vi "Example UI.TestLauncher.vi"() -> ()   [LabVIEW 2016, in "Instrument.PPMS2 UI.lvclass"]
doc: "JKI State Machine Objects (SMO) 1.0.0.5\nJKI - JKI\nCopyright (c) 2016, JKI"
uses:
  Instrument.PPMS2 UI.lvclass
  C:/Program Files (x86)/National Instruments/LabVIEW 2016/vi.lib/JKI/JKI SMO/SMO/SMO.lvclass
  C:/Program Files (x86)/National Instruments/LabVIEW 2016/vi.lib/JKI/JKI SMO/SMO.UI/SMO.UI.lvclass
  instrument.PPMS2/instrument.PPMS2.lvclass
  C:/Program Files (x86)/National Instruments/LabVIEW 2016/user.lib/LevyLab/Levylab Instruments/SMOs/Instrument/Instrument.lvclass
  <vilib>/JKI/JKI SMO/SMO/Typedefs/SMOState --Enum.ctl
  <vilib>/JKI/JKI SMO/SMO/SMO.lvclass
  <vilib>/JKI/JKI SMO/SMO.UI/SMO.UI.lvclass
panel:
  out "error out":errorcluster
  in  "Stop":bool
  # "SMO UI Test Launcher"
  # "For instructions on how to use the JKI State Machine Objects, examples and video tutorials, visit:\nhttp://jki.net/state-machine-objects/\n\nJKI State Machine Objects™\nhttp://jki.net/state-machine-objects/\nCopyright (C) 2005-2015, JKI <info@jki.net>\nALL RIGHTS RESERVED"
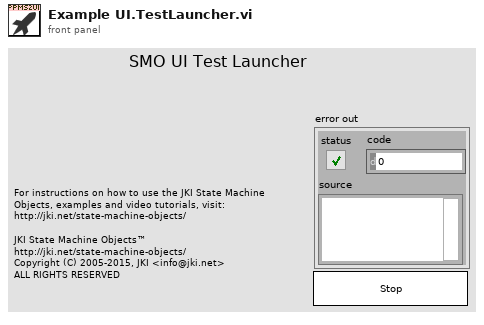
[diagram p1: front panel]
types:
  T1 = typedef "SMO.lvclass/Public Events.ctl" = cluster{"Error":refnum<user-event>, "State":refnum<user-event>, "Reserve State":refnum<user-event>}
  T2 = typedef "SMO.UI.lvclass/PublicEvents--Cluster.ctl" = cluster{"UI Hidden":refnum<user-event>, "UI State":refnum<user-event>}
  T3 = typedef "SMO.lvclass/SMOState --Enum.ctl" = enum16{"unknown", "Created", "Started", "Stopped"}
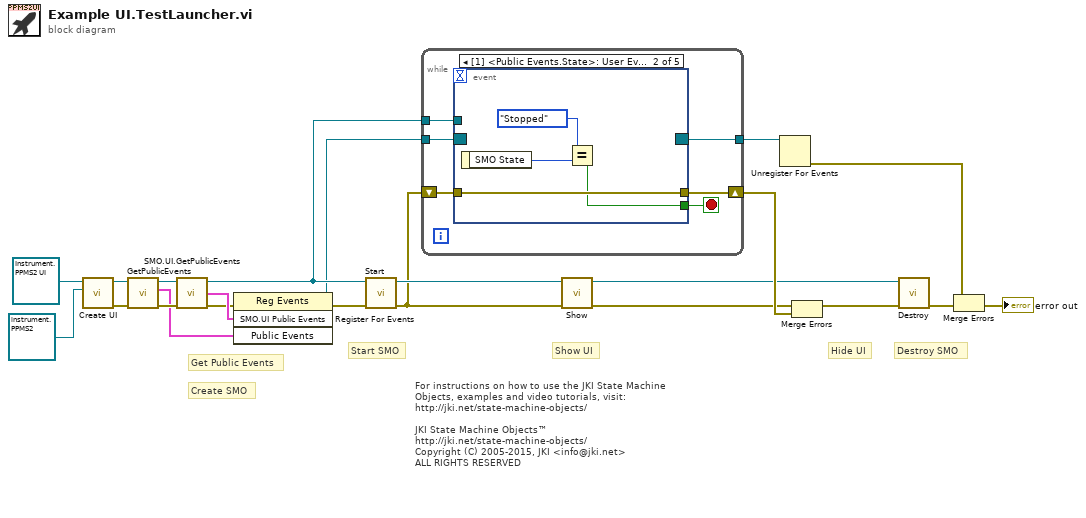
[diagram p0: block diagram]
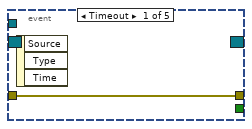
[diagram p2: hidden frame]
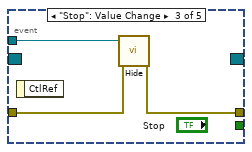
[diagram p3: hidden frame]
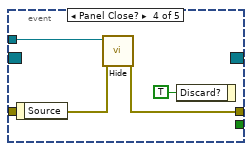
[diagram p4: hidden frame]
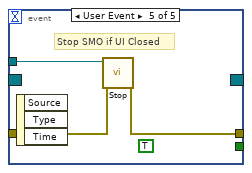
[diagram p5: hidden frame]
diagram:
  # "Hide UI"
  # "Show UI"
  # "For instructions on how to use the JKI State Machine Objects, examples and video tutorials, visit:\nhttp://jki.net/state-machine-objects/\n\nJKI State Machine Objects™\nhttp://jki.net/state-machine-objects/\nCopyright (C) 2005-2015, JKI <info@jki.net>\nALL RIGHTS RESERVED"
  # "Get Public Events"
  # "Start SMO"
  # "Destroy SMO"
  # "Create SMO"
  n1 = call "Create UI.vi"("Instrument.Example in"=refnum<class "instrument.PPMS2.lvclass"> refnum ("instrument.PPMS2.lvclass"), "Instrument.Example UI in"=refnum<class "Instrument.PPMS2 UI.lvclass"> refnum ("SMO.Template.lvclass")) -> ("error out"=w4:errorcluster, "Instrument.Example UI out"=w3:refnum<class "Instrument.PPMS2 UI.lvclass">)  [unwired: 8 in]
  n2 = call <vilib>:"GetPublicEvents.vi"("error in (no error)"=w4, "SMO"=w3) -> ("error out"=w6:errorcluster, "Public Events"=w5:T1, "SMO out"=w7:refnum<class "Instrument.PPMS2 UI.lvclass">)  [unwired: 7 in]
  n3 = call <vilib>:"SMO.UI.GetPublicEvents.vi"("error in (no error)"=w6, "SMO.UI"=w7) -> ("error out"=w10:errorcluster, "SMO.UI Public Events"=w11:T2, "SMO.UI out"=w12:refnum<class "Instrument.PPMS2 UI.lvclass">)  [unwired: 7 in]
  n4 = register-events(error in=w10, w11, w5) -> (reference out=w8:refnum<event-registration>, error out=w9:errorcluster)  [unwired: 1 in]
  n5 = call <vilib>:"Start.vi"("error in (no error)"=w9, "SMO"=w12) -> ("error out"=w16:errorcluster, "SMO out"=w17:refnum<class "Instrument.PPMS2 UI.lvclass">)  [unwired: 8 in]
  n6 = while {
    shift-right: [w27] -> w21
    shift-left: w16 -> [w26]
    tunnel: w8 -> [w25]
    tunnel: [w24] -> w22
    tunnel: w12 -> [w23]
    stop <- w28 stop-if-true
    n7 = event shown="[1] <Public Events.State>: User Event" {
      selector: w25 -> [_ _ _ _ _]
      dyn-events: [_ _ _ _ _] -> w24
      timeout: _ -> [_ _ _ _ _]
      tunnel: [_ w30 _ _ _] -> w28
      tunnel: w23 -> [_ _ w36 w39 w43]
      tunnel: [w29 w33 w34 w37 w42] -> w27
      tunnel: w26 -> [w29 w33 w35 w38 w41]
      event Timeout {
        n8 = event-data() -> ()  [unwired: 1 in, 3 out]
      }
      event User Event {
        n9 = event-data() -> ("SMO State"=w32:T3)  [unwired: 1 in]
        n10 = Equal?(x=SMOState_--Enum."Stopped", y=w32) -> (x = y?=w30:bool)
      }
      event "Stop": Value Change {
        n11 = event-data() -> ()  [unwired: 1 in, 1 out]
        n12 = call <vilib>:"Hide.vi"("error in (no error)"=w35, "SMO.UI"=w36) -> ("error out"=w34:errorcluster)  [unwired: 8 in, 1 out]
      }
      event Panel Close? {
        n13 = event-data() -> ()  [unwired: 1 in, 1 out]
        n14 = call <vilib>:"Hide.vi"("error in (no error)"=w38, "SMO.UI"=w39) -> ("error out"=w37:errorcluster)  [unwired: 8 in, 1 out]
        n15 = event-data("Discard?"=TRUE ("OK")) -> ()  [unwired: 1 in, 1 out]
      }
      event User Event {
        (unwired) TRUE ("OK")
        # "Stop SMO if UI Closed"
        n16 = event-data() -> ()  [unwired: 1 in, 3 out]
        n17 = call <vilib>:"Stop.vi"("error in (no error)"=w41, "SMO"=w43) -> ("error out"=w42:errorcluster)  [unwired: 8 in, 1 out]
      }
    }
  }
  n18 = call <vilib>:"Show.vi"("error in (no error)"=w16, "SMO.UI"=w17) -> ("error out"=w15:errorcluster, "SMO.UI out"=w14:refnum<class "Instrument.PPMS2 UI.lvclass">)  [unwired: 8 in]
  n19 = Unregister For Events(event registration refnum=w22) -> (error out=w20:errorcluster)  [unwired: 1 in]
  n20 = Merge Errors(w15, w21) -> (w13:errorcluster)
  n21 = call <vilib>:"Destroy.vi"("error in (no error)"=w13, "SMO"=w14) -> ("error out"=w18:errorcluster)  [unwired: 9 in]
  n22 = Merge Errors(w20, w18) -> (→"error out":errorcluster)
